vi "dump.vi"(8 "error in (no error)":errorcluster, 10 "indent":T1, 11 "self in":refnum<class "Identifier.lvclass">) -> (0 "error out":errorcluster, 2 "mlir":string, 3 "self out":refnum<class "Identifier.lvclass">)   [LabVIEW 2020, in "mlir.lvlib" / "Identifier.lvclass"]
uses:
  Identifier.lvclass
  Node/indent.ctl
  mlir.lvlib
panel:
  # "Dumps the AST node and its children in MLIR format."
  # "String representing the AST in MLIR."
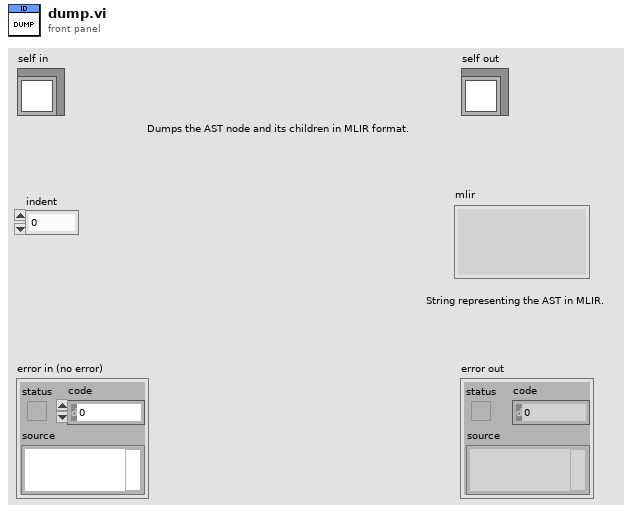
[diagram p1: front panel]
types:
  T1 = typedef "mlir.lvlib/indent.ctl" = u32
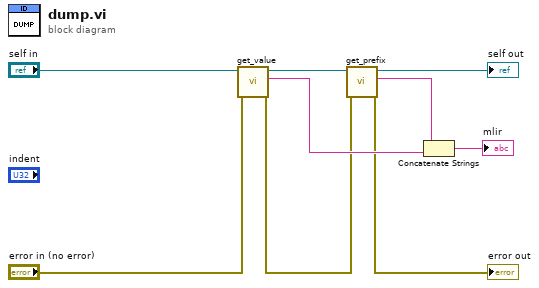
[diagram p0: block diagram]
diagram:
  n1 = call-dynamic "get_value.vi"("error in (no error)"="error in (no error)", "Identifier in"="self in") -> ("error out"=w2:errorcluster, "value"=w4:string, "Identifier out"=w5:refnum<class "Identifier.lvclass">)  [unwired: 7 in]
  n2 = call "get_prefix.vi"("error in (no error)"=w2, "self in"=w5) -> ("error out"=→"error out":errorcluster, "_prefix_"=w7:string, "self out"=→"self out":refnum<class "Identifier.lvclass">)  [unwired: 7 in]
  n3 = Concatenate Strings(w7, w4) -> (→"mlir":string)
